vi "Util_Convert String to Time Stamp.vi"(11 "Time":string) -> (3 "Time":timestamp format="%<%I:%M:%S %p\n%x>T")   [LabVIEW 2013]
uses:
  <vilib>/Utility/miscctls.llb/LVDateTimeRec.ctl
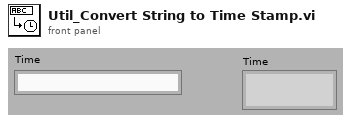
[diagram p1: front panel]
types:
  T1 = typedef "LVDateTimeRec.ctl" = cluster{"fractional second":dbl, "second":i32, "minute":i32, "hour":i32, "day of month":i32, "month":i32, "year":i32, "day of week":i32, "day of year":i32, "DST":i32}
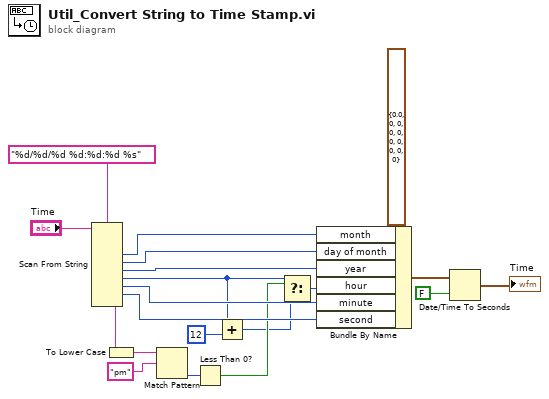
[diagram p0: block diagram]
diagram:
  n1 = Scan From String(format string="%d/%d/%d %d:%d:%d %s", input string="Time") -> (output 1=w15:i32, output 2=w14:i32, output 3=w13:i32, output 4=w3:i32, output 5=w12:i32, output 6=w11:i32, output 7=w10:string)  [unwired: 2 in, 10 out]
  n2 = To Lower Case(string=w10) -> (all lower case string=w9:string)
  n3 = Match Pattern(string=w9, regular expression="pm") -> (offset past match=w7:i32)  [unwired: 4 out]
  n4 = Less Than 0?(x=w7) -> (x < 0?=w4:bool)
  n5 = Add(x=w3, y=12) -> (x+y=w2:i32)
  n6 = Select(t=w3, s=w4, f=w2) -> (s? t:f=w5:i32)
  n7 = Bundle By Name(cluster=T1 {"fractional second"=0.0, "second"=0, "minute"=0, "hour"=0, "day of month"=0, "month"=0, "year"=0, "day of week"=0, "day of year"=0, "DST"=0} ("date time rec"), "month"=w15, "day of month"=w14, "year"=w13, "hour"=w5, "minute"=w12, "second"=w11) -> (w18:T1)
  n8 = Date/Time To Seconds(1:FALSE ("is UTC (F)"), 2:w18) -> (0:→"Time":timestamp)
